vi "6 ch resopnance scanner (FPGA) fixed pix clock.vi"() -> ()   [LabVIEW 2012]
uses:
  <vilib>/eio/EIONode/EIONode.xnode
  <vilib>/rvi/eio/common/nirviEmuTemplateMethod_errors.vi
  <vilib>/rvi/DataTransferAndStorage/Container/XNode/niFpgaContainer.xnode
  <vilib>/rvi/interface/RandomDataEmulation/nirviRandomDataFpgaReadWriteTemplate.vi
  <vilib>/platform/TimedLoop/XDataNode/XDataNode.xnode
  <vilib>/Platform/TimedLoop/XDataNode/nitl_modes.ctl
  <vilib>/Platform/TimedLoop/XDataNode/XDNodeRunTimeDep.lvlib
  <vilib>/Platform/TimedLoop/XDataNode/wakeup.ctl
  <vilib>/Platform/TimedLoop/XDataNode/timing_clust.ctl
panel:
  in  "lines at once":i16=4999
  in  "dwell time in ticks":i32
  in  "samples per half period":i16=4999
  in  "Start Delay (Ticks)":i16 caption="Start delay (Ticks)"
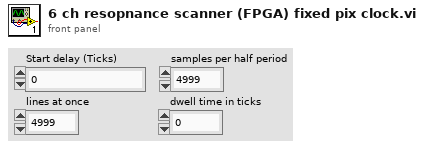
[diagram p1: front panel]
types:
  T1 = cluster{"IO Module\\AI A0":i32, "IO Module\\AI A1":i32, "IO Module\\AI A1 2":i32, "IO Module\\AI A1 3":i32, "IO Module\\AI A1 4":i32, "IO Module\\AI A1 5":i32}
  T2 = typedef "XDNodeRunTimeDep.lvlib/timing_clust.ctl" = cluster{"Expected End [f-1]":u64, "Actual End [f-1]":u64, "Finished Late? [f-1]":bool, "Expected End [i-1]":u64, "Actual End [i-1]":u64, "Finished Late? [i-1]":bool, "Expected Start [i]":u64, "Actual Start [i]":u64, "Expected Start [f]":u64, "Actual Start [f]":u64, "Source Name":string, "Structure Name":string, "Period":i64, "Deadline":i64, "Offset":i64, "Start":i64, "Priority":i32, "Timeout":i32, "Mode":T3, "Wakeup Reason":T4, "Error":errorcluster, "Source Type":string, "Secondary Source Type":string, "Global End Time":u64, "Global Start Time":u64, "Frame Duration":u64, "Iteration Duration":u64, "Assigned CPU":i32, "I/O Scan Engine Mode":u32}
  T3 = typedef "XDNodeRunTimeDep.lvlib/nitl_modes.ctl" = enum32{"No Change", "Process missed periods, maintain original phase", "Discard missed periods, maintain original phase", "Process missed periods, ignore original phase", "Discard missed periods, ignore original phase"}
  T4 = typedef "XDNodeRunTimeDep.lvlib/wakeup.ctl" = enum32{"Normal", "Aborted", "Asynchronous wakeup", "Timing source error", "Timed loop error", "Timeout"}
  T5 = cluster{"IO Module\\AI A0":i16, "IO Module\\AI A1":i16, "IO Module\\AI A2":i16, "IO Module\\AI A3":i16, "IO Module\\AI A4":i16, "IO Module\\AI A5":i16}
  T6 = cluster{"IO Module\\AI A0":i32, "IO Module\\AI A1":i32, "IO Module\\AI A2":i32, "IO Module\\AI A3":i32, "IO Module\\AI A4":i32, "IO Module\\AI A5":i32}
  T7 = cluster{"IO Module\\AI A0":i32, "IO Module\\AI A1":i32, i32, i32, i32, i32}
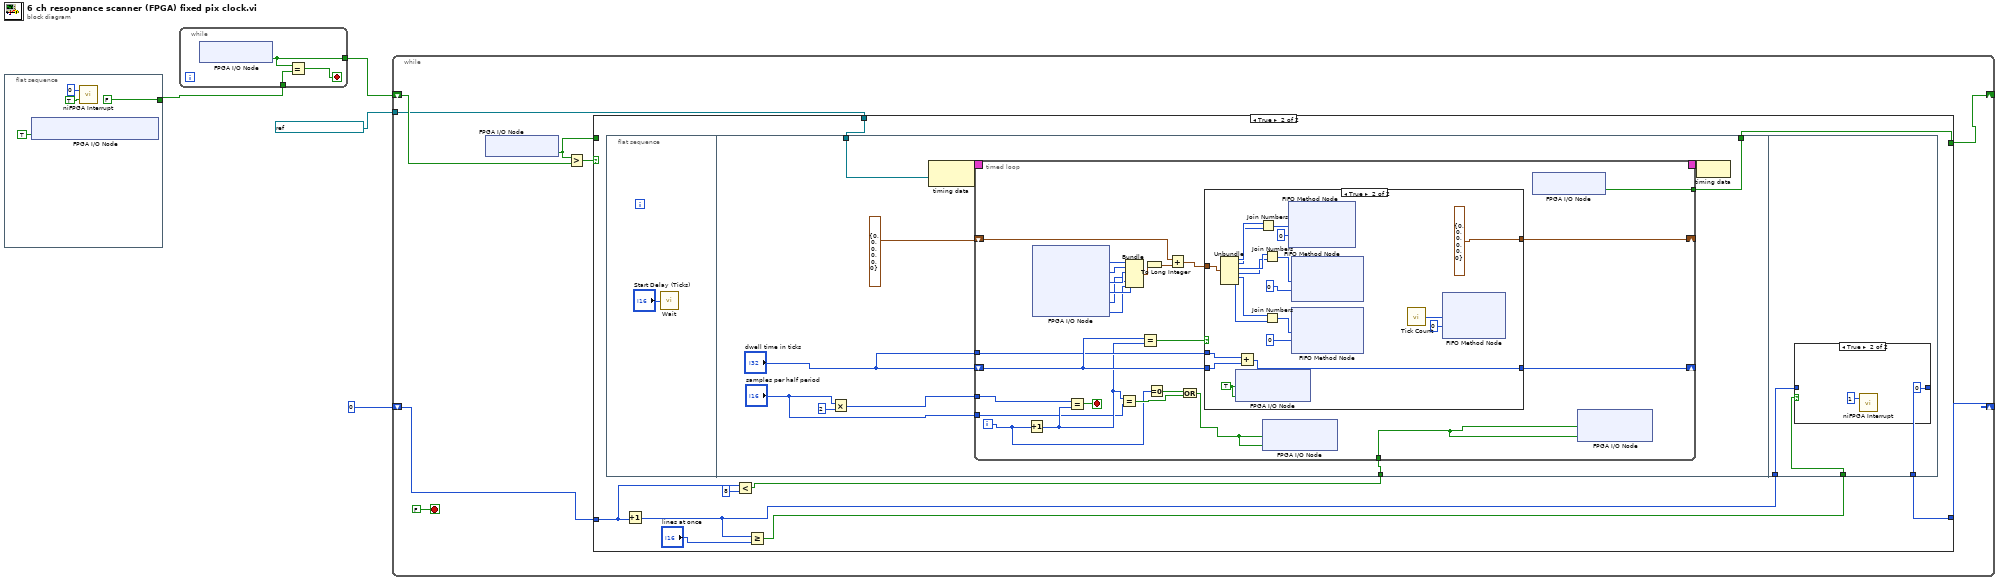
[diagram p0: block diagram]
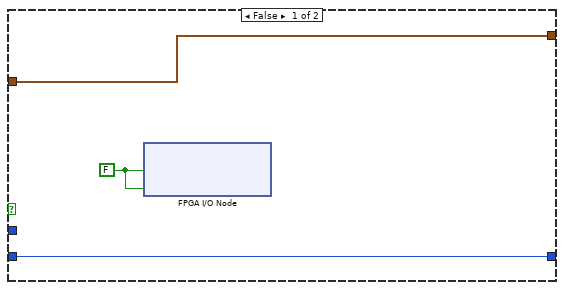
[diagram p3: hidden frame]
diagram:
  n1 = flat-sequence {
    tunnel: [FALSE ("IO Module\\DI 0")] -> w2
    frame #0 {
      n2 = xnode "FPGA I/O Node"("IO Module\\Digital Output Enable"=TRUE ("IO Module\\Digital Output Enable")) -> ()  [unwired: 1 in, 1 out]
      n3 = call <vilib>:"niFPGA Interrupt.vi"("Wait Until Cleared (F)"=TRUE, "IRQ Number (0)"=u8 0) -> ()  [unwired: 1 in]
    }
  }
  n4 = while {
    tunnel: w2 -> [w11]
    tunnel: [w9] -> w1
    stop <- w10 stop-if-true
    n5 = xnode "FPGA I/O Node"() -> ("IO Module\\DI 0"=w9:bool)  [unwired: 1 in, 1 out]
    n6 = Equal?(x=w9, y=w11) -> (x = y?=w10:bool)
  }
  n7 = while {
    shift-right: [w18] -> _
    shift-left: w1 -> [w19]
    shift-right: [w16] -> _
    shift-left: i16 0 ("IRQ Number (0)") -> [w15]
    tunnel: refnum<k21> "40 MHz Onboard Clock" ("Source Name") -> [w13]
    stop <- FALSE stop-if-true
    n8 = xnode "FPGA I/O Node"() -> ("IO Module\\DI 0"=w12:bool)  [unwired: 1 in, 1 out]
    n9 = Greater?(x=w12, y=w19) -> (0:w14:bool)
    n10 = case shown="True" w14 {
      tunnel: [w20 w22] -> w18
      tunnel: w15 -> [w21 w24]
      tunnel: [w21 w28] -> w16
      tunnel: w13 -> [_ w27]
      tunnel: w12 -> [w20 _]
      frame False {
      }
      frame True {
        n11 = flat-sequence {
          tunnel: w27 -> [w37]
          tunnel: w26 -> [w33]
          tunnel: [w32] -> w22
          tunnel: w30 -> [w98]
          tunnel: w29 -> [w97]
          tunnel: [w96] -> w28
          frame #0 {
            n12 = call "Wait"("Count(Ticks)"="Start Delay (Ticks)") -> ()  [unwired: 1 out]
          }
          frame #1 {
            n13 = Multiply(x="samples per half period", y=i16 2) -> (x*y=w35:i16)
            n14 = node-c288(w37) -> (w39:T2)
            n15 = timed-loop {
              tunnel: w35 -> [w65]
              shift-right: [w56] -> _
              shift-left: T1 {"IO Module\\AI A0"=0, "IO Module\\AI A1"=0, "IO Module\\AI A1 2"=0, "IO Module\\AI A1 3"=0, "IO Module\\AI A1 4"=0, "IO Module\\AI A1 5"=0} ("x+y") -> [w61]
              shift-right: [w59] -> _
              shift-left: "dwell time in ticks" -> [w55]
              tunnel: "dwell time in ticks" -> [w54]
              timing: w39 -> [_]
              timing-out: [_] -> w38
              tunnel: "samples per half period" -> [w45]
              tunnel: w33 -> [w51]
              tunnel: [w44] -> w32
              i -> [w47]
              stop <- w66 stop-if-true
              n16 = Increment(x=w47) -> (x+1=w46:i32)
              n17 = xnode "FPGA I/O Node"() -> ("IO Module\\AI A0"=w64:i16, "IO Module\\AI A1"=w63:i16, "IO Module\\AI A2"=w53:i16, "IO Module\\AI A3"=w52:i16, "IO Module\\AI A4"=w43:i16, "IO Module\\AI A5"=w42:i16)  [unwired: 6 in, 6 out]
              n18 = Equal?(x=w65, y=w46) -> (x = y?=w66:bool)
              n19 = Equal?(x=w46, y=w45) -> (x = y?=w49:bool)
              n20 = Bundle("IO Module\\AI A0"=w64, "IO Module\\AI A1"=w63, "IO Module\\AI A2"=w53, "IO Module\\AI A3"=w52, "IO Module\\AI A4"=w43, "IO Module\\AI A5"=w42) -> (w57:T5)  [unwired: 1 in]
              n21 = Equal?(x=w55, y=w46) -> (x = y?=w58:bool)
              n22 = To Long Integer(number=w57) -> (32bit integer=w62:T6)
              n23 = Equal To 0?(x=w47) -> (x = 0?=w50:bool)
              n24 = Add(x=w61, y=w62) -> (x+y=w60:T7)
              n25 = Or(x=w50, y=w49) -> (x .or. y?=w48:bool)
              n26 = case shown="True" w58 {
                tunnel: w60 -> [w69 w87]
                tunnel: [w69 T1 {"IO Module\\AI A0"=0, "IO Module\\AI A1"=0, "IO Module\\AI A1 2"=0, "IO Module\\AI A1 3"=0, "IO Module\\AI A1 4"=0, "IO Module\\AI A1 5"=0} ("x+y")] -> w56
                tunnel: [w68 w80] -> w59
                tunnel: w55 -> [w68 w81]
                tunnel: w54 -> [_ w82]
                frame False {
                  w67 = FALSE ("IO Module\\D0 0")
                  n27 = xnode "FPGA I/O Node"("IO Module\\D0 0"=w67, "PXI_Trig0"=w67) -> ()  [unwired: 2 in, 2 out]
                }
                frame True {
                  w75 = TRUE ("IO Module\\D0 0")
                  n28 = Unbundle(w87) -> ("IO Module\\AI A0"=w86:i32, "IO Module\\AI A1"=w85:i32, w79:i32, w78:i32, w74:i32, w73:i32)
                  n29 = xnode "FPGA I/O Node"("IO Module\\D0 0"=w75, "PXI_Trig0"=w75) -> ()  [unwired: 2 in, 2 out]
                  n30 = Add(x=w82, y=w81) -> (x+y=w80:i32)
                  n31 = Join Numbers(hi=w86, lo=w85) -> ((hi.lo)=w89:u64)
                  n32 = Join Numbers(hi=w79, lo=w78) -> ((hi.lo)=w76:u64)
                  n33 = Join Numbers(hi=w74, lo=w73) -> ((hi.lo)=w72:u64)
                  n34 = xnode ("FIFO Method Node")("Element"=w89, "Timeout"=0) -> ()  [unwired: 1 in, 2 out]
                  n35 = xnode ("FIFO Method Node")("Element"=w76, "Timeout"=0) -> ()  [unwired: 1 in, 2 out]
                  n36 = xnode ("FIFO Method Node")("Element"=w72, "Timeout"=0) -> ()  [unwired: 1 in, 2 out]
                  n37 = call "Tick Count"() -> ("Tick Count(Ticks)"=w83:u32)
                  n38 = xnode ("FIFO Method Node")("Element"=w83, "Timeout"=0) -> ()  [unwired: 1 in, 2 out]
                }
              }
              n39 = xnode "FPGA I/O Node"("IO Module\\D0 1"=w48, "PXI_Trig1"=w48) -> ()  [unwired: 2 in, 2 out]
              n40 = xnode "FPGA I/O Node"() -> ("IO Module\\DI 0"=w44:bool)  [unwired: 1 in, 1 out]
              n41 = xnode "FPGA I/O Node"("PXI_Trig2"=w51, "IO Module\\D0 2"=w51) -> ()  [unwired: 2 in, 2 out]
            }
            n42 = node-c288(w38) -> ()
          }
          frame #2 {
            n43 = case shown="True" w97 {
              tunnel: w98 -> [w99 _]
              tunnel: [w99 u8 0] -> w96
              frame False {
              }
              frame True {
                n44 = call <vilib>:"niFPGA Interrupt.vi"("IRQ Number (0)"=u8 1) -> ()  [unwired: 2 in]
              }
            }
          }
        }
        n45 = Increment(x=w24) -> (x+1=w30:i16)
        n46 = Less?(x=w24, y=i16 8) -> (x < y?=w26:bool)
        n47 = Greater Or Equal?(x=w30, y="lines at once") -> (x >= y?=w29:bool)
      }
    }
  }
